vi "Get Window GWL_Style.vi"(8 "error in (no error)":errorcluster, 11 "Hwnd":u32) -> (0 "error out":errorcluster, 3 "Style":u32)   [LabVIEW 2011]
doc: "This VI will read the GWL_Style for a given window <B>Hwnd</B>."
uses:
  user32.dll
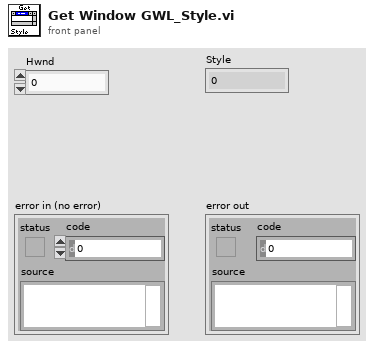
[diagram p1: front panel]
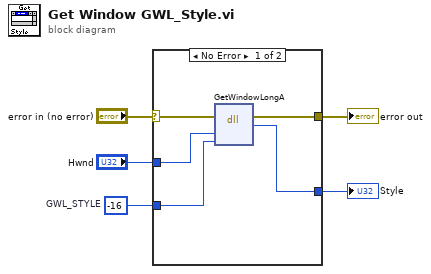
[diagram p0: block diagram]
diagram:
  w5 = -16  # GWL_STYLE
  n1 = case shown="No Error" "error in (no error)" {
    selector: "error in (no error)" -> [w7 w11]
    tunnel: w5 -> [w10 _]
    tunnel: "Hwnd" -> [w9 _]
    tunnel: [w8 w11] -> w3
    tunnel: [w6 _] -> w1
    frame No Error {
      n2 = dll-call lib="user32.dll" fn="GetWindowLongA" ("SetParent")(error in=w7, "Hwnd"=w9, "Index"=w10) -> (error out=w8:errorcluster, "return type"=w6:u32)  [unwired: 4 in, 1 out]
    }
    frame Error {
    }
  }
  "error out" <- w3
  "Style" <- w1
